vi "Toggle.vi"(11 "Button":bool) -> (3 "Output":bool)   [LabVIEW 2015]
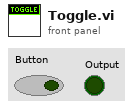
[diagram p1: front panel]
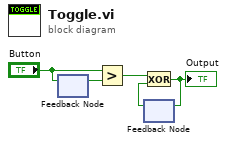
[diagram p0: block diagram]
diagram:
  n1 = feedback-in #1("Button") -> ()
  n2 = feedback #1() -> (w4:bool)  [unwired: 1 in]
  n3 = Greater?(x="Button", y=w4) -> (0:w3:bool)
  n4 = feedback #2() -> (w1:bool)  [unwired: 1 in]
  n5 = Exclusive Or(1:w1, 2:w3) -> (0:w2:bool)
  "Output" <- w2
  n6 = feedback-in #2(w2) -> ()
